vi "Check Cache Type.vi"(8 "error in (no error)":errorcluster, 11 "Processing In":refnum<class "Processing.lvclass">) -> (0 "error out":errorcluster, 2 "Request Cache Type":T1, 4 "Value":string)   [LabVIEW 2020, in "HTTP Server.lvlib" / "Caching.lvclass"]
uses:
  Caching.lvclass
  Processing/Processing.lvclass
  Request Cache Type.ctl
  HTTP Server.lvlib
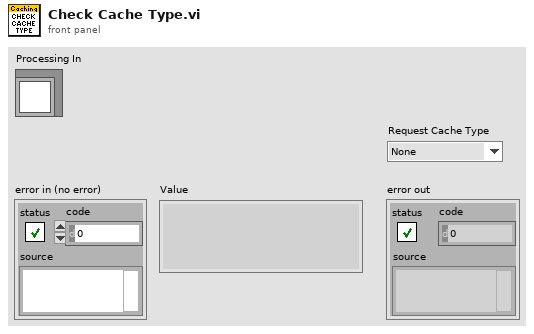
[diagram p1: front panel]
types:
  T1 = typedef "HTTP Server.lvlib/Request Cache Type.ctl" = enum16{"None", "Modified", "ETag", "Expires"}
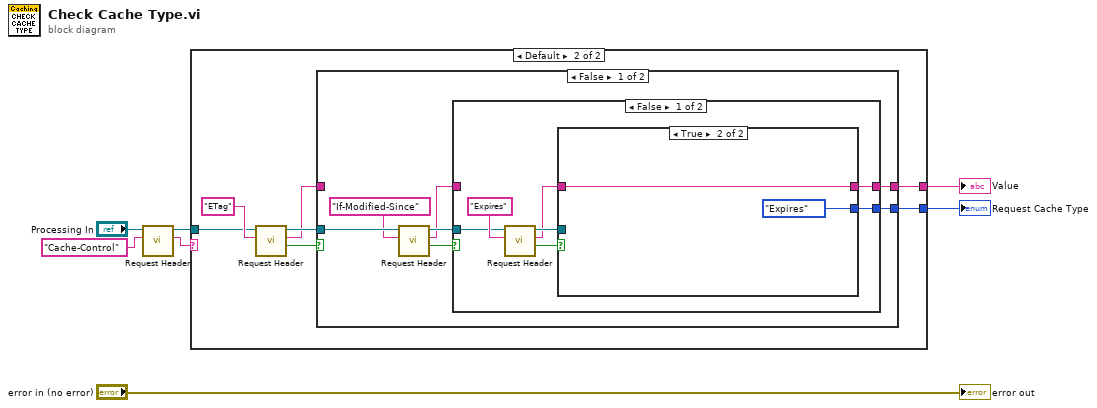
[diagram p0: block diagram]
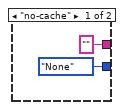
[diagram p2: hidden frame]
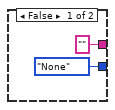
[diagram p3: hidden frame]
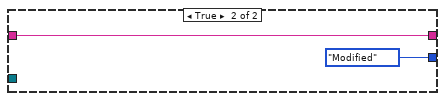
[diagram p4: hidden frame]
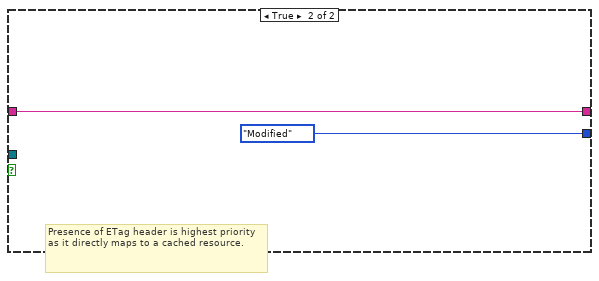
[diagram p5: hidden frame]
diagram:
  n1 = call "Request Header.vi"("Header"="Cache-Control", "Processing in"="Processing In") -> ("Value"=w1:string, "Processing out"=w2:refnum<class "Processing.lvclass">)  [unwired: 6 in, 2 out]
  n2 = case shown="Default" w1 {
    tunnel: [Request_Cache_Type."None" ("Request Cache Type") w13] -> w6
    tunnel: ["" ("Value") w11] -> w5
    tunnel: w2 -> [_ w10]
    frame "no-cache" {
    }
    frame Default {
      n3 = call "Request Header.vi"("Header"="ETag", "Processing in"=w10) -> ("Exists"=w15:bool, "Value"=w12:string, "Processing out"=w14:refnum<class "Processing.lvclass">)  [unwired: 6 in, 1 out]
      n4 = case shown="False" w15 {
        tunnel: w14 -> [w23 _]
        tunnel: [w19 Request_Cache_Type."Modified" ("Request Cache Type")] -> w13
        tunnel: w12 -> [_ w37]
        tunnel: [w18 w37] -> w11
        frame False {
          n5 = call "Request Header.vi"("Header"="If-Modified-Since", "Processing in"=w23) -> ("Exists"=w21:bool, "Value"=w17:string, "Processing out"=w20:refnum<class "Processing.lvclass">)  [unwired: 6 in, 1 out]
          n6 = case shown="False" w21 {
            tunnel: w20 -> [w29 _]
            tunnel: [w26 Request_Cache_Type."Modified" ("Request Cache Type")] -> w19
            tunnel: [w25 w35] -> w18
            tunnel: w17 -> [_ w35]
            frame False {
              n7 = call "Request Header.vi"("Header"="Expires", "Processing in"=w29) -> ("Exists"=w28:bool, "Value"=w24:string, "Processing out"=w27:refnum<class "Processing.lvclass">)  [unwired: 6 in, 1 out]
              n8 = case shown="True" w28 {
                tunnel: w27 -> [_ _]
                tunnel: [Request_Cache_Type."None" ("Request Cache Type") Request_Cache_Type."Expires" ("Request Cache Type")] -> w26
                tunnel: ["" ("Value") w33] -> w25
                tunnel: w24 -> [_ w33]
                frame False {
                }
                frame True {
                }
              }
            }
            frame True {
            }
          }
        }
        frame True {
          # "Presence of ETag header is highest priority as it directly maps to a cached resource."
        }
      }
    }
  }
  "Request Cache Type" <- w6
  "Value" <- w5
  "error out" <- "error in (no error)"
